vi "TMP36SensorSubVI.vi"(1 "Raw Input (V)":dbl) -> (0 "Temperature (C)":dbl)   [LabVIEW 2016]
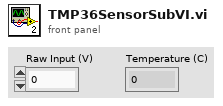
[diagram p1: front panel]
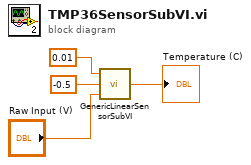
[diagram p0: block diagram]
diagram:
  n1 = call "GenericLinearSensorSubVI.vi"("Raw Input"="Raw Input (V)", "Offset"=-0.5 ("Offset (V)"), "Slope"=0.01 ("Slope (V/C)")) -> ("Scaled Output"=→"Temperature (C)":dbl)
